vi "Do.vi"(8 "error in (no error)":errorcluster, 10 "Actor in":refnum<class "Actor.lvclass">, 11 "New Command Status Msg":refnum<class "New Command Status Msg.lvclass">) -> (0 "error out":errorcluster, 2 "Actor out":refnum<class "Actor.lvclass">)   [LabVIEW 2013, in "Command Processor.lvlib" / "New Command Status Msg.lvclass"]
doc: "This VI delivers the message to the actor by calling the appropriate method(s) on the actor."
uses:
  New Command Status Msg.lvclass
  Command Processor/Command Processor.lvclass
  <vilib>/ActorFramework/Actor/Actor.lvclass
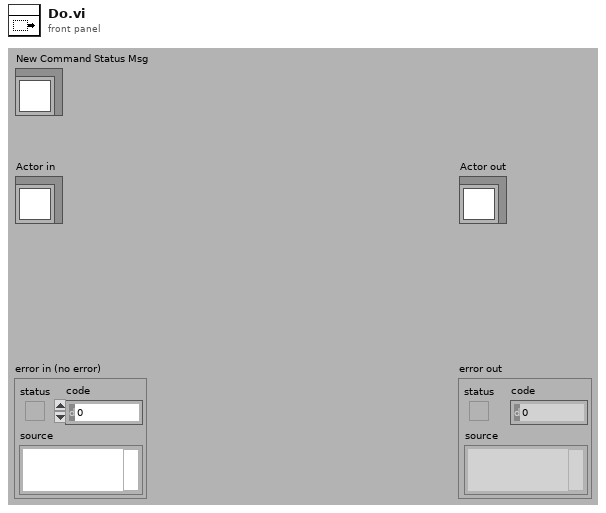
[diagram p1: front panel]
types:
  T1 = typedef "Command Processor.lvlib/Command.lvlib/Command.lvclass/Command Status.ctl" = cluster{"Command Name":string, "Current State Status":T2, "Command Start Time":timestamp, "Command End Time":timestamp, "Previous State Status":T2}
  T2 = typedef "Command Processor.lvlib/Command.lvlib/Command.lvclass/State Status.ctl" = cluster{"State Name":string, "State Entry Time":timestamp, "State Exit Time":timestamp}
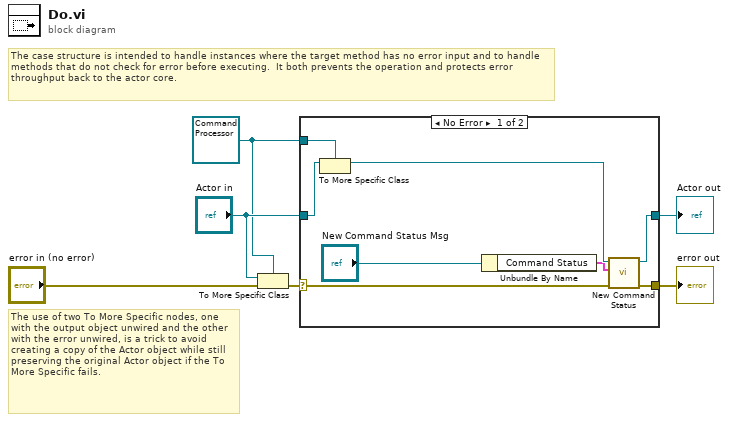
[diagram p0: block diagram]
diagram:
  w1 = refnum<class "Command Processor.lvclass"> refnum ("Actor in")
  # "The use of two To More Specific nodes, one with the output object unwired and the other with the error unwired, is a trick to avoid creating a copy of the Actor object while still preserving the original Actor object if the To More Specific fails."
  # "The case structure is intended to handle instances where the target method has no error input and to handle methods that do not check for error before executing.  It both prevents the operation and protects error throughput back to the actor core."
  n1 = To More Specific Class(target class=w1, reference="Actor in", error in="error in (no error)") -> (error out=w5:errorcluster)  [unwired: 1 out]
  n2 = case shown="No Error" w5 {
    selector: w5 -> [w12 w16]
    tunnel: [w14 w16] -> w4
    tunnel: [w13 w15] -> w3
    tunnel: "Actor in" -> [w11 w15]
    tunnel: w1 -> [w10 _]
    frame No Error {
      n3 = To More Specific Class(target class=w10, reference=w11) -> (specific class reference=w9:refnum<class "Command Processor.lvclass">)  [unwired: 1 in, 1 out]
      n4 = Unbundle By Name("New Command Status Msg") -> ("Command Status"=w7:T1)
      n5 = call-dynamic "New Command Status.vi"("error in (no error)"=w12, "Command Status"=w7, "Command Processor in"=w9) -> ("error out"=w14:errorcluster, "Command Processor out"=w13:refnum<class "Command Processor.lvclass">)  [unwired: 7 in]
    }
    frame Error {
      # "If type check fails, pass the original object out again."
    }
  }
  "error out" <- w4
  "Actor out" <- w3
